vi "readTriggerXML.vi"(8 "error in (no error)":errorcluster, 10 "NativeXML in":refnum<class "NativeXML.lvclass">, 11 "WinX32Settings in":refnum<class "WinX32Settings.lvclass">) -> (0 "error out":errorcluster, 2 "NativeXML out":refnum<class "NativeXML.lvclass">, 3 "WinX32Settings out":refnum<class "WinX32Settings.lvclass">)   [LabVIEW 2011, in "Tools.lvlib" / "Settings.lvlib" / "WinX32Settings.lvclass"]
uses:
  WinX32Settings.lvclass
  NativeXML/NativeXML.lvclass
  WinX32Settings.lvclass/WinX32Settings.ctl
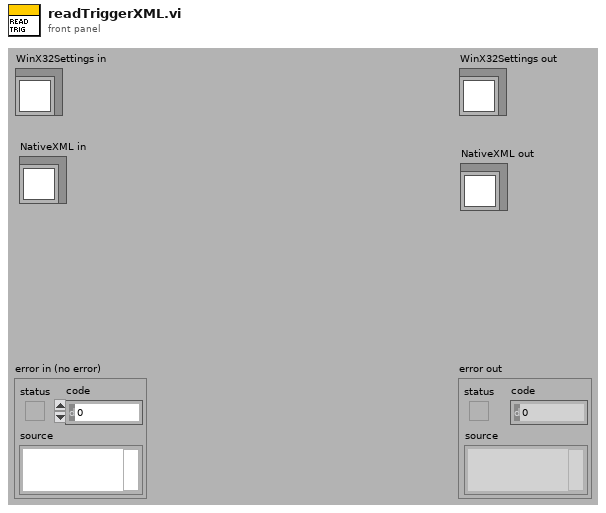
[diagram p1: front panel]
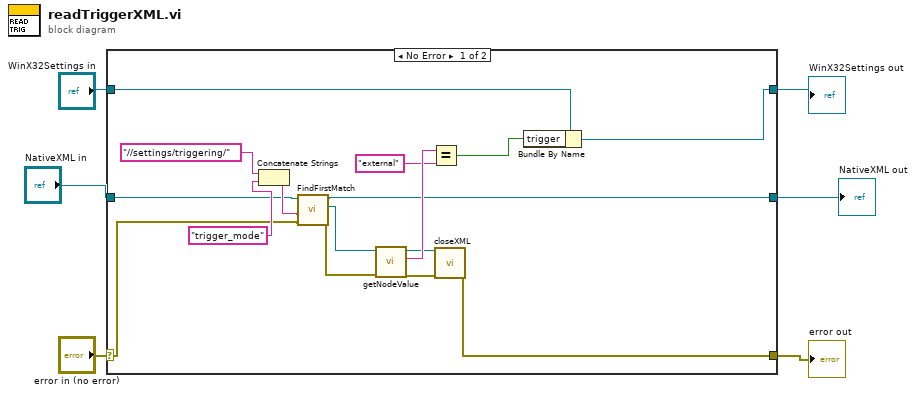
[diagram p0: block diagram]
diagram:
  n1 = case shown="No Error" "error in (no error)" {
    selector: "error in (no error)" -> [w9 w23]
    tunnel: [w15 w23] -> w3
    tunnel: [w19 w24] -> w4
    tunnel: "WinX32Settings in" -> [w20 w24]
    tunnel: "NativeXML in" -> [w7 w25]
    tunnel: [w12 w25] -> w1
    frame No Error {
      n2 = Concatenate Strings("//settings/triggering/" ("searchElementIn"), "trigger_mode") -> (w8:string)
      n3 = call "FindFirstMatch.vi"("error in (no error)"=w9, "xPath"=w8, "NativeXML in"=w7) -> ("error out"=w10:errorcluster, "NativeXML match"=w11:refnum<class "NativeXML.lvclass">, "NativeXML out"=w12:refnum<class "NativeXML.lvclass">)  [unwired: 6 in]
      n4 = call "getNodeValue.vi"("error in (no error)"=w10, "NativeXML in"=w11) -> ("error out"=w16:errorcluster, "Value"=w22:string, "NativeXML out"=w17:refnum<class "NativeXML.lvclass">)  [unwired: 7 in]
      n5 = Equal?(x=w22, y="external") -> (x = y?=w18:bool)
      n6 = call "closeXML.vi"("error in (no error)"=w16, "NativeXML in"=w17) -> ("error out"=w15:errorcluster)  [unwired: 9 in]
      n7 = Bundle By Name(cluster=w20, "trigger"=w18) -> (w19:refnum<class "WinX32Settings.lvclass">)
    }
    frame Error {
    }
  }
  "error out" <- w3
  "WinX32Settings out" <- w4
  "NativeXML out" <- w1
